vi "Display ViewableActors.vi"(8 "error in (no error)":errorcluster, 10 "ViewableActor Enqueuers":refnum<class "Message Enqueuer.lvclass">[](array[class]), 11 "SubPanel Grid View in":refnum<class "SubPanel Grid View.lvclass">) -> (0 "error out":errorcluster, 3 "SubPanel Grid View out":refnum<class "SubPanel Grid View.lvclass">)   [LabVIEW 2012, in "Win8uiDemo.lvlib" / "SubPanel Grid View.lvclass"]
uses:
  SubPanel Grid View.lvclass
  <vilib>/ActorFramework/Message Enqueuer/Message Enqueuer.lvclass
  SubPanel Grid View.lvclass/SubPanel Grid View.ctl
  Win8uiFramework/Insert Into SubPanel Msg.lvclass/Insert Into SubPanel Msg.ctl
  <vilib>/ActorFramework/Message Enqueuer/Message Enqueuer.lvclass/Message Enqueuer.ctl
  SubPanel 3x3 View/Read SubPanel Array.vi
  Write ViewableActor Enqueuers.vi
  <vilib>/ActorFramework/Message Enqueuer/Enqueue.vi
  <vilib>/ActorFramework/Message Priority Queue/Priority Enqueue.vi
  Win8uiFramework/Insert Into SubPanel Msg.lvclass
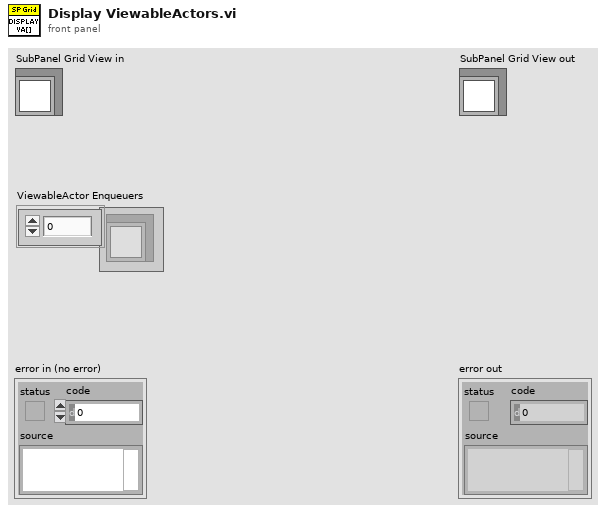
[diagram p1: front panel]
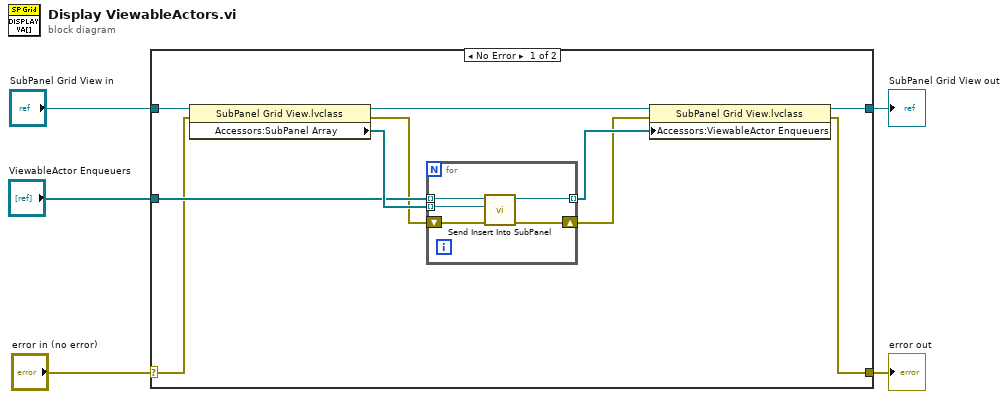
[diagram p0: block diagram]
diagram:
  n1 = case shown="No Error" "error in (no error)" {
    selector: "error in (no error)" -> [w10 w22]
    tunnel: [w6 w22] -> w4
    tunnel: [w9 w21] -> w2
    tunnel: "SubPanel Grid View in" -> [w15 w21]
    tunnel: "ViewableActor Enqueuers" -> [w12 _]
    frame No Error {
      n2 = property class="SubPanel Grid View.lvclass"(reference=w15, error in=w10) -> (reference out=w14:refnum<class "SubPanel Grid View.lvclass">, error out=w11:errorcluster, "Accessors:SubPanel Array"=w13:refnum<vi>[])
      n3 = for {
        tunnel: w13 -> [w20] mode=indexing
        tunnel: w12 -> [w19] mode=indexing
        shift-right: [w17] -> w7
        shift-left: w11 -> [w18]
        tunnel: [w16] -> w8 mode=indexing
        n4 = call "Send Insert Into SubPanel.vi"("error in (no error)"=w18, "SubPanel Ref"=w20, "Message Enqueuer"=w19) -> ("error out"=w17:errorcluster, "Message Enqueuer out"=w16:refnum<class "Message Enqueuer.lvclass">)  [unwired: 7 in]
      }
      n5 = property class="SubPanel Grid View.lvclass"(reference=w14, error in=w7, "Accessors:ViewableActor Enqueuers"=w8) -> (reference out=w9:refnum<class "SubPanel Grid View.lvclass">, error out=w6:errorcluster)
    }
    frame Error {
    }
  }
  "error out" <- w4
  "SubPanel Grid View out" <- w2
